vi "ziDisconnectDevice.vi"(8 "Error In":errorcluster, 10 "Device Serial":string, 11 "Handle In":T1 {"Handle" format="0x%08x"; "Conn" format="0x%08x"}) -> (0 "Error Out":errorcluster, 3 "Handle Out":T1 {"Handle" format="0x%08x"; "Conn" format="0x%08x"})   [LabVIEW 2009, in "Zurich Instruments LabOne.lvlib"]
uses:
  <instrlib>/Zurich Instruments LabOne/Zurich Instruments LabOne.lvlib
  <instrlib>/Zurich Instruments LabOne/Public/ziTypeHandle.ctl
  <instrlib>/Zurich Instruments LabOne/Private/ziLV32.dll
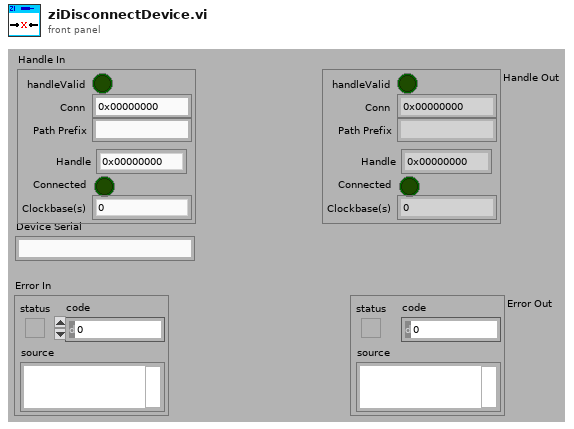
[diagram p1: front panel]
types:
  T1 = typedef "Zurich Instruments LabOne.lvlib/ziTypeHandle.ctl" = cluster{"handleValid":bool, "Conn":u64, "Path Prefix":string, "Handle":u64, "Connected":bool, "Clockbase(s)":dbl}
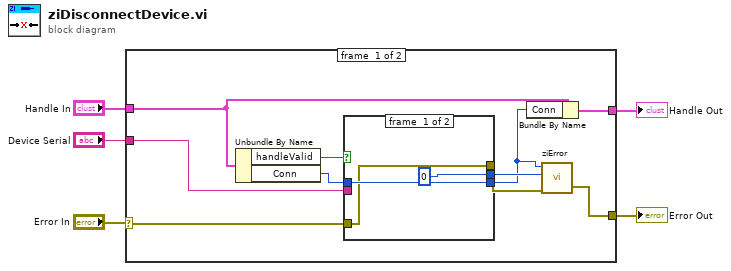
[diagram p0: block diagram]
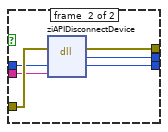
[diagram p2: hidden frame]
diagram:
  n1 = case shown="No Error" "Error In" {
    selector: "Error In" -> [w9 w26]
    tunnel: [w14 w26] -> w5
    tunnel: [w10 w25] -> w4
    tunnel: "Handle In" -> [w7 w25]
    tunnel: "Device Serial" -> [w8 _]
    frame #0 {
      n2 = Unbundle By Name(w7) -> ("handleValid"=w11:bool, "Conn"=w15:u64)
      n3 = case shown="True" w11 {
        tunnel: w9 -> [w17 w24]
        tunnel: w15 -> [w18 w23]
        tunnel: w8 -> [_ w22]
        tunnel: [w17 w21] -> w13
        tunnel: [u32 0 ("return type") w20] -> w12
        tunnel: [w18 w19] -> w6
        frame #0 {
        }
        frame #1 {
          n4 = dll-call lib="C:/Program Files (x86)/National Instruments/LabVIEW 2009/instr.lib/Zurich Instruments LabOne/Private/ziLV*.*" fn="ziAPIDisconnectDevice"(error in=w24, "Conn"=w23, "deviceSerial"=w22) -> (error out=w21:errorcluster, "return type"=w20:u32, "Conn"=w19:u64)  [unwired: 3 in, 1 out]
        }
      }
      n5 = Bundle By Name(cluster=w7, "Conn"=w6) -> (w10:T1)
      n6 = call <instrlib>:"ziError.vi"("Conn"=w6, "ziErrorCode"=w12, "Error In"=w13) -> ("Error Out"=w14:errorcluster)  [unwired: 2 in, 1 out]
    }
    frame #1 {
    }
  }
  "Error Out" <- w5
  "Handle Out" <- w4
